vi "ManipulateModuleName.vi"(0 "ModuleListArrayIn":string[](array[string])=["AcPwr.PPS", "AcPwr.Chroma"], 5 "MatchExpression":string="[.]", 9 "ModuleListSingleEntry":string="AcPwr.PPS") -> (3 "ModuleListArrayOut":string[](array[string])=["AcPwr.PPS", "AcPwr.Chroma"], 4 "AfterMatch:ModuleListArray":string[](array[string]), 6 "BeforeMatch:ModuleListArray":string[](array[string]), 8 "BeforeMatchWithoutRedundantEntries:ModuleListArray":string[](array[string]), 10 "BeforeMatch:ModuleListSingleEntry":string, 15 "AfterMatch:ModuleListSingleEntry":string)   [LabVIEW 2018, in "Test.lvclass"]
doc: "This VI seperates out the [xxx] and [yyy] from the input \"yyy.xxx\". Where xxx is the type name and yyy is the module name. This function is helpful when using multiple types of the same module."
uses:
  Test.lvclass
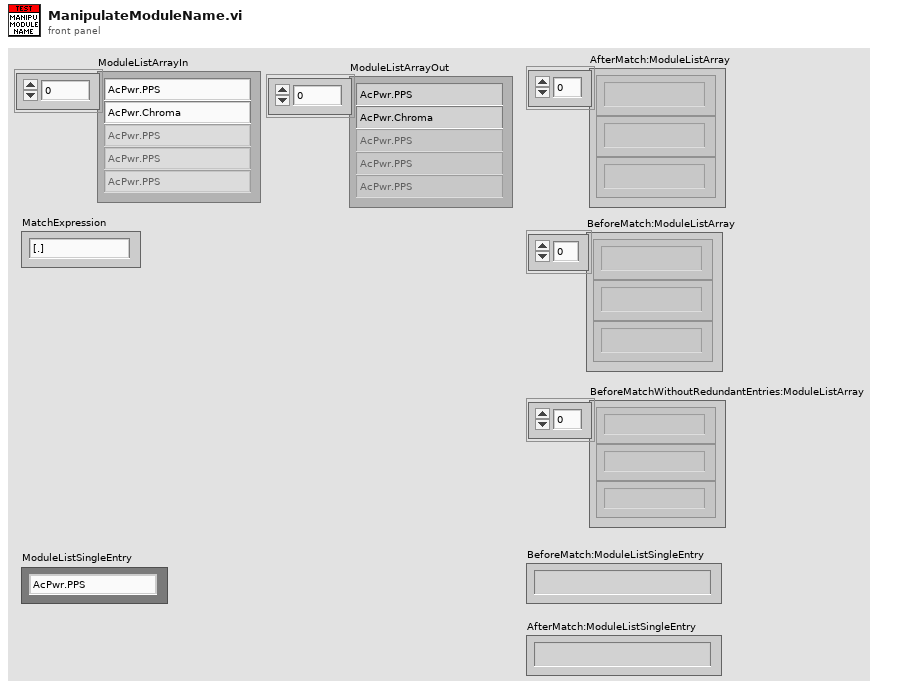
[diagram p1: front panel]
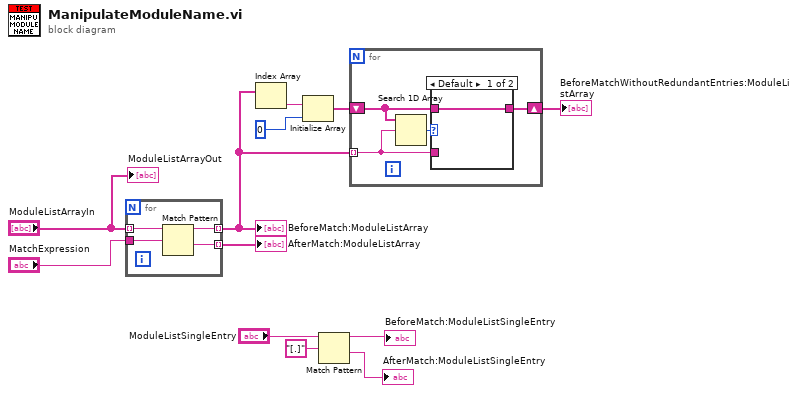
[diagram p0: block diagram]
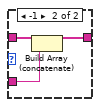
[diagram p2: hidden frame]
diagram:
  n1 = for {
    tunnel: "ModuleListArrayIn" -> [w16] mode=indexing
    tunnel: [w15] -> w6 mode=indexing
    tunnel: [w14] -> w8 mode=indexing
    tunnel: "MatchExpression" -> [w13]
    n2 = Match Pattern(string=w16, regular expression=w13) -> (before substring=w15:string, after substring=w14:string)  [unwired: 1 in, 2 out]
  }
  "BeforeMatch:ModuleListArray" <- w6
  "AfterMatch:ModuleListArray" <- w8
  n3 = Index Array(array=w6) -> (element=w9:string)  [unwired: 1 in]
  n4 = Initialize Array(w9, 0 ("Dimension Size")) -> (w10:string[])
  n5 = Match Pattern(string="ModuleListSingleEntry", regular expression="[.]") -> (before substring=→"BeforeMatch:ModuleListSingleEntry":string, after substring=→"AfterMatch:ModuleListSingleEntry":string)  [unwired: 1 in, 2 out]
  n6 = for {
    tunnel: w6 -> [w19] mode=indexing
    shift-right: [w18] -> w7
    shift-left: w10 -> [w17]
    n7 = Search 1D Array(1D array=w17, element=w19) -> (index of element=w20:i32)  [unwired: 1 in]
    n8 = case shown="Default" w20 {
      tunnel: w19 -> [_ w24]
      tunnel: [w21 w22] -> w18
      tunnel: w17 -> [w21 w23]
      frame Default {
      }
      frame -1 {
        n9 = Build Array (concatenate)(w23, w24) -> (w22:string[])
      }
    }
  }
  "BeforeMatchWithoutRedundantEntries:ModuleListArray" <- w7
  "ModuleListArrayOut" <- "ModuleListArrayIn"
